vi "Get BLISS_Copy Selected Images.vi"(6 "Size":string, 7 "BLISS Type":enum16{"Reject Images", "PBQA Images"}(ring), 8 "error in (no error)":errorcluster, 9 "View":string, 10 "base path":path, 11 "Data Parameters in":T1) -> (0 "error out":errorcluster, 1 "Data Parameters Out":T1)   [LabVIEW 2020]
uses:
  MC5e Gobal_Variables.vi
  MC5e Squad_Info.ctl
  MC5e Data_Parameters.ctl
  MC5e Unit_Status_List.ctl
  MC5e Terrain types.ctl
  Location.ctl
  MC5e Unit.ctl
  MC5e Force.ctl
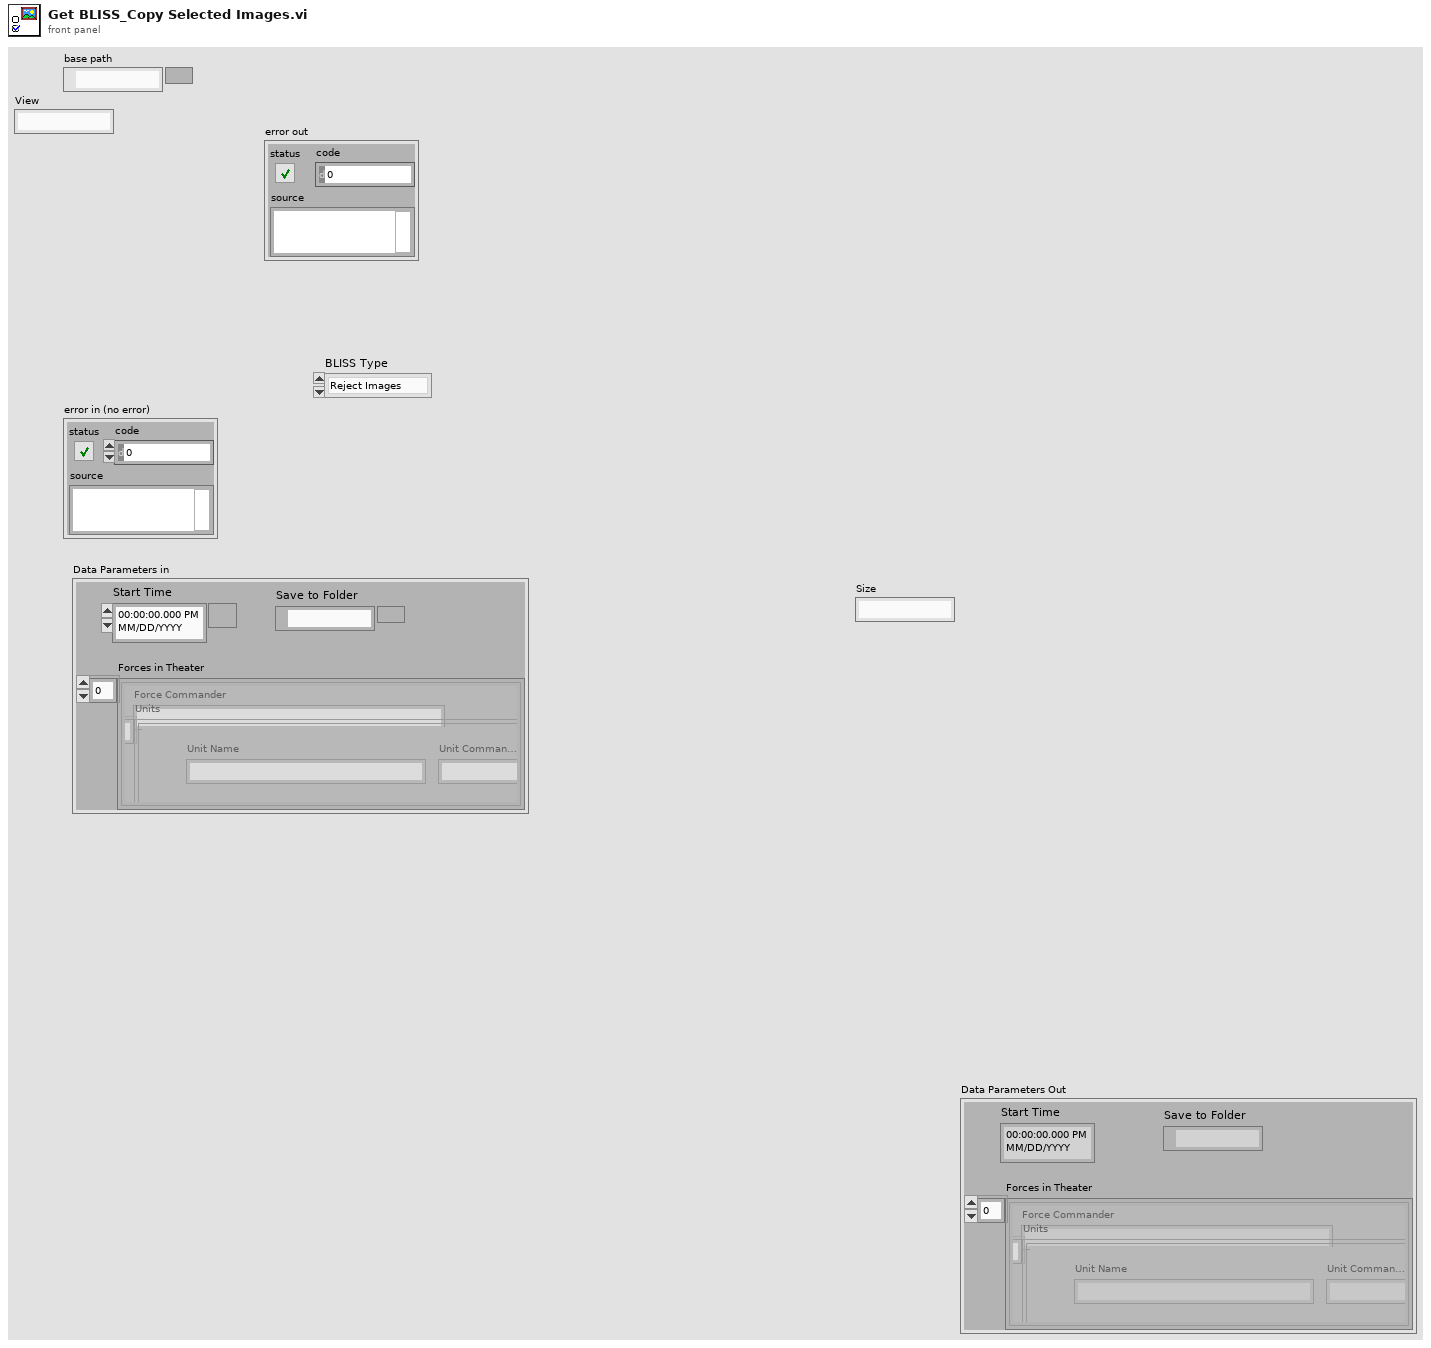
[diagram p1: front panel]
types:
  T1 = typedef "MC5e Data_Parameters.ctl" = cluster{"Start Time":timestamp, "Save to Folder":path, "Forces in Theater":T2[]}
  T2 = typedef "MC5e Force.ctl" = cluster{"Force Commander":string, "Units":T3[]}
  T3 = typedef "MC5e Unit.ctl" = cluster{"Squad List":T4, "Unit Fatigue Level":enum16{"Not Fatigued", "Fatigued", "Seriously Fatigued"}, "Flying Unit":bool, "Mounted Unit":bool, "Difficult Terrain Types":T6, "Full BR":dbl, "Defending from Stronghold":bool, "Speed":dbl, "Capacity %":dbl, "Morale":dbl, "Current BR":dbl, "Location":T7, "Unit Name":string, "Unit Commander":string, "Unit Notes":string}
  T4 = typedef "MC5e Unit_Status_List.ctl" = T5[]
  T5 = typedef "MC5e Squad_Info.ctl" = cluster{"Squad Name":string, "# Soldiers":dbl, "Battle Rating":dbl, "Flying":bool, "Mounted":bool, "Speed":dbl, "Range":dbl, "Morale":dbl, "Token Image":variant, "Max Endurance":dbl, "Current Endurance":dbl, "Difficult Terrain":T6}
  T6 = typedef "MC5e Terrain types.ctl" = cluster{"Artic / snow / ice)":bool, "Coast":bool, "Desert / sand":bool, "Forest / woodland":bool, "Grassland / plains":bool, "Mountain / canyons":bool, "Underdark / caverns":bool, "Acquatic / rivers, lakes, ocean":bool}
  T7 = typedef "Location.ctl" = cluster{"X coordinate":dbl, "Y coordinate":dbl}
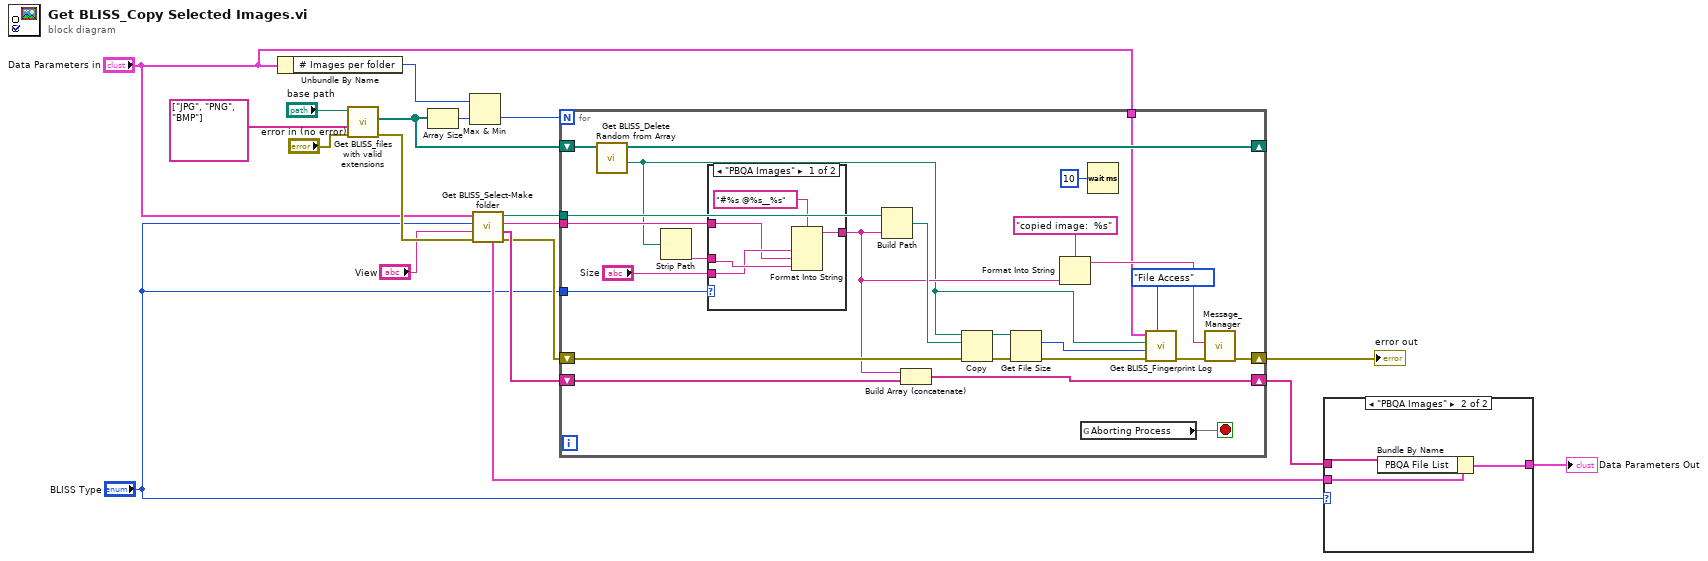
[diagram p0: block diagram]
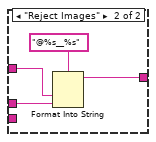
[diagram p2: hidden frame]
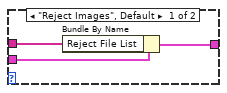
[diagram p3: hidden frame]
diagram:
  n1 = Unbundle By Name("Data Parameters in") -> ("# Images per folder"=w18:i32)
  n2 = call "Get BLISS_files with valid extensions.vi"("error in (no error)"="error in (no error)", "extensions"=string[] ["JPG", "PNG", "BMP"], "path in"="base path") -> ("error out"=w8:errorcluster, "valid filepaths"=w13:path[])  [unwired: 6 in, 1 out]
  n3 = Array Size(array=w13) -> (size(s)=w14:i32)
  n4 = Max & Min(x=w18, y=w14) -> (min(x,y)=w15:i32)  [unwired: 1 out]
  n5 = call "Get BLISS_Select-Make folder.vi"("error in (no error)"=w8, "View"="View", "BLISS Type"="BLISS Type", "Data Parameters in in"="Data Parameters in") -> ("error out"=w7:errorcluster, "File List"=w17:string[], "Server Name"=w6:string, "dup path"=w9:path, "Data Parameters out"=w4:T1)  [unwired: 3 in]
  n6 = for {
    N: w15 -> [_]
    shift-right: [w35] -> w11
    shift-left: w7 -> [w43]
    shift-right: [w41] -> _
    shift-left: w13 -> [w42]
    shift-right: [w39] -> w16
    shift-left: w17 -> [w40]
    tunnel: w9 -> [w38]
    tunnel: w6 -> [w32]
    tunnel: "BLISS Type" -> [w30]
    tunnel: "Data Parameters in" -> [w25]
    stop <- w37 stop-if-true
    n7 = call "Get BLISS_Delete Random from Array.vi"("filepath array in"=w42) -> ("random deleted filepath"=w24:path, "remaining array"=w41:path[])  [unwired: 9 in]
    n8 = Strip Path(path=w24) -> (name=w31:string)  [unwired: 1 out]
    n9 = case shown="\"PBQA Images\"" w30 {
      tunnel: [w48 w52] -> w26
      tunnel: w32 -> [w45 w51]
      tunnel: w31 -> [w47 w50]
      tunnel: "Size" -> [w46 _]
      frame "PBQA Images" {
        n10 = Format Into String(format string="#%s @%s__%s", w46, w45, w47) -> (resulting string=w48:string)  [unwired: 2 in, 1 out]
      }
      frame "Reject Images" {
        n11 = Format Into String(format string="@%s__%s", w51, w50) -> (resulting string=w52:string)  [unwired: 2 in, 1 out]
      }
    }
    n12 = Build Path(base path=w38, name or relative path=w26) -> (appended path=w44:path)
    n13 = Build Array (concatenate)(w26, w40) -> (w39:string[])
    n14 = Copy(8:w43, 10:w44, 11:w24) -> (0:w23:errorcluster, 3:w21:path)  [unwired: 2 in, 1 out]
    n15 = Get File Size(file=w21, error in=w23) -> (size (in bytes)=w20:i64, 0:w22:errorcluster)  [unwired: 1 out]
    n16 = Format Into String(format string="copied image:  %s", w26) -> (resulting string=w34:string)  [unwired: 2 in, 1 out]
    n17 = global read "MC5e Gobal_Variables.vi" "Aborting Process"() -> (w37)
    n18 = Wait (ms)(milliseconds to wait=u32 10) -> ()  [unwired: 1 out]
    n19 = call "Get BLISS_Fingerprint Log.vi"("Action"=enum16{"Server Access", "File Access"}."File Access", "error in (no error)"=w22, "size (in bytes)"=w20, "source filepath"=w24, "Data Parameters in"=w25) -> ("error out"=w27:errorcluster)  [unwired: 6 in]
    n20 = call "Message_Manager.vi"("error in"=w27, "New Entry"=w34) -> ("error out"=w35:errorcluster)  [unwired: 4 in, 5 out]
  }
  "error out" <- w11
  n21 = case shown="\"PBQA Images\"" "BLISS Type" {
    tunnel: w4 -> [w56 w57]
    tunnel: w16 -> [w55 w59]
    tunnel: [w54 w58] -> w10
    frame "Reject Images", Default {
      n22 = Bundle By Name(cluster=w56, "Reject File List"=w55) -> (w54:T1)
    }
    frame "PBQA Images" {
      n23 = Bundle By Name(cluster=w57, "PBQA File List"=w59) -> (w58:T1)
    }
  }
  "Data Parameters Out" <- w10
